vi "Acquire Data.vi"(8 "Error In":errorcluster, 11 "LHW-Aquisition-Actor in":refnum<class "LHW-Aquisition-Actor.lvclass">) -> (0 "Error Out":errorcluster, 3 "LHW-Aquisition-Actor out":refnum<class "LHW-Aquisition-Actor.lvclass">)   [LabVIEW 2014, in "LHW-Acquisition.lvlib" / "LHW-Aquisition-Actor.lvclass"]
doc: "Acquire Data."
uses:
  LHW-Aquisition-Actor.lvclass
  LHW-Aquisition-Actor.lvclass/LHW-Aquisition-Actor.ctl
  <vilib>/ActorFramework/Actor/Actor.lvclass/Actor.ctl
  LHW-GUI-Actor Messages/Update LHW Data Msg/Update LHW Data Msg.lvclass/Update LHW Data Msg.ctl
  <vilib>/ActorFramework/Message Enqueuer/Message Enqueuer.lvclass/Message Enqueuer.ctl
  <vilib>/ActorFramework/Message Enqueuer/Enqueue.vi
  <vilib>/ActorFramework/Message Priority Queue/Priority Enqueue.vi
  <vilib>/ActorFramework/Message Enqueuer/Message Enqueuer.lvclass
  LHW-GUI-Actor Messages/Update LHW Data Msg/Update LHW Data Msg.lvclass
  <vilib>/ActorFramework/Actor/Actor.lvclass
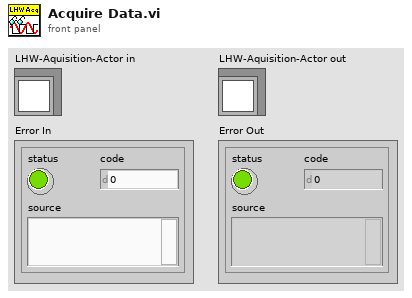
[diagram p1: front panel]
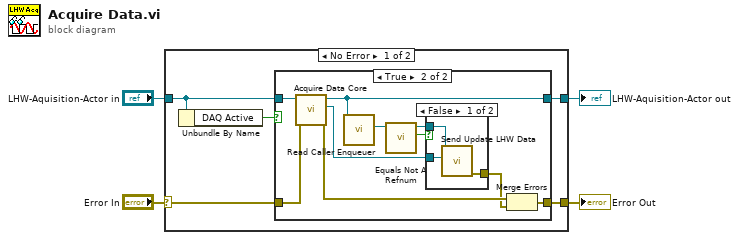
[diagram p0: block diagram]
diagram:
  n1 = case shown="No Error" "Error In" {
    selector: "Error In" -> [w7 w25]
    tunnel: [w6 w25] -> w3
    tunnel: [w8 w24] -> w1
    tunnel: "LHW-Aquisition-Actor in" -> [w9 w24]
    frame No Error {
      n2 = Unbundle By Name(w9) -> ("DAQ Active"=w5:bool)
      n3 = case shown="True" w5 {
        tunnel: w9 -> [w11 w20]
        tunnel: [w11 w18] -> w8
        tunnel: w7 -> [w10 w19]
        tunnel: [w10 w16] -> w6
        frame False {
        }
        frame True {
          n4 = call-dynamic "Acquire Data Core.vi"("Error In"=w19, "LHW-Aquisition-Actor in"=w20) -> ("Error Out"=w15:errorcluster, "LHW-Data"=w17:refnum<class "LHW-Data.lvclass">, "LHW-Aquisition-Actor out"=w18:refnum<class "LHW-Aquisition-Actor.lvclass">)  [unwired: 7 in]
          n5 = call <vilib>:"Read Caller Enqueuer.vi"("Actor"=w18) -> ("Caller Enqueuer"=w13:refnum<class "Message Enqueuer.lvclass">)  [unwired: 10 in]
          n6 = call <vilib>:"Equals Not A Refnum.vi"("Message Enqueuer"=w13) -> ("Not a refnum?"=w12:bool)  [unwired: 10 in]
          n7 = case shown="False" w12 {
            tunnel: w17 -> [w23 _]
            tunnel: [w22 _] -> w14
            tunnel: w13 -> [w21 _]
            frame False {
              n8 = call "Send Update LHW Data.vi"("LHW-Data"=w23, "Message Enqueuer"=w21) -> ("error out"=w22:errorcluster)  [unwired: 8 in, 1 out]
            }
            frame True {
            }
          }
          n9 = Merge Errors(w15, w14) -> (w16:errorcluster)
        }
      }
    }
    frame Error {
    }
  }
  "Error Out" <- w3
  "LHW-Aquisition-Actor out" <- w1
